vi "Get_Dev_SN.vi"(8 "error in (no error)":errorcluster) -> (0 "error out":errorcluster, 1 "dev":tag[](array[tag]), 2 "Dev_SN 2":string[](array[string]), 3 "Dev_SN":u32[](array[numeric]) format="%.0x")   [LabVIEW 2015]
uses:
  <resource>/objmgr/daqmx.rc
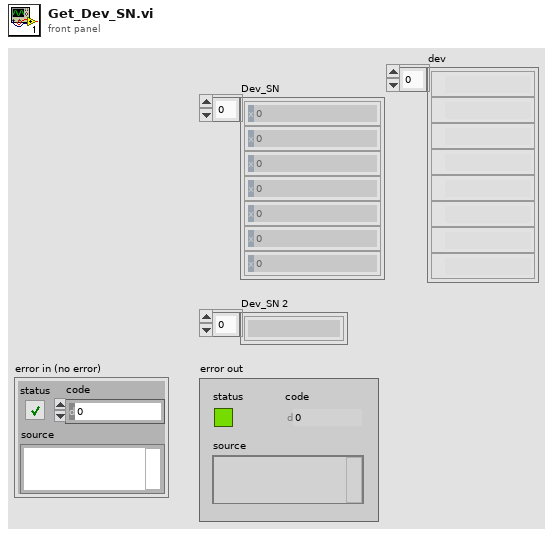
[diagram p1: front panel]
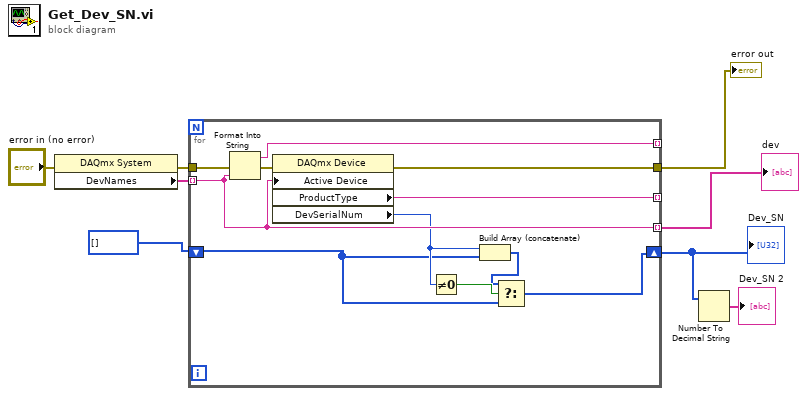
[diagram p0: block diagram]
diagram:
  n1 = property class="DAQmx System"(error in="error in (no error)") -> (error out=w3:errorcluster, "DevNames"=w2:tag[])  [unwired: 1 in, 1 out]
  n2 = for {
    tunnel: w2 -> [w17] mode=indexing
    tunnel: [w19] -> _ mode=indexing
    tunnel: [w18] -> _ mode=indexing
    tunnel: [w17] -> w1 mode=indexing
    tunnel: w3 -> [w15]
    tunnel: [w14] -> w4
    shift-right: [w9] -> w7
    shift-left: u32[] [] ("Dev_SN 2") -> [w11]
    n3 = Format Into String(error in=w15, w17) -> (resulting string=w18:string, error out=w16:errorcluster)  [unwired: 2 in]
    n4 = property class="DAQmx Device"(error in=w16, "Active Device"=w17) -> (error out=w14:errorcluster, "ProductType"=w19:string, "DevSerialNum"=w12:u32)  [unwired: 1 in, 1 out]
    n5 = Not Equal To 0?(x=w12) -> (x != 0?=w13:bool)
    n6 = Build Array (concatenate)(w12, w11) -> (w10:u32[])
    n7 = Select(t=w10, s=w13, f=w11) -> (s? t:f=w9:u32[])
  }
  "error out" <- w4
  "Dev_SN" <- w7
  "dev" <- w1
  n8 = Number To Decimal String(number=w7) -> (decimal integer string=→"Dev_SN 2":string[])  [unwired: 1 in]
